vi "GetProperties.vi"(8 "error in":errorcluster, 11 "GObject in":refnum<class "GObject.lvclass">) -> (0 "error out":errorcluster, 3 "GObject out":refnum<class "GObject.lvclass">)   [LabVIEW 2014, in "GObject.lvclass"]
uses:
  GObject.lvclass
  GObject.lvclass/GObject.ctl
  Generic/Generic.lvclass
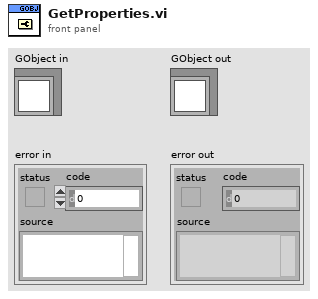
[diagram p1: front panel]
types:
  T1 = typedef "LVBoundsTypeDef.ctl" = cluster{"Width":u32, "Height":u32}
  T2 = typedef "LVRectTypeDef.ctl" = cluster{"Left":i16, "Top":i16, "Right":i16, "Bottom":i16}
  T3 = typedef "LVPositionTypeDef.ctl" = cluster{"Left":i32, "Top":i32}
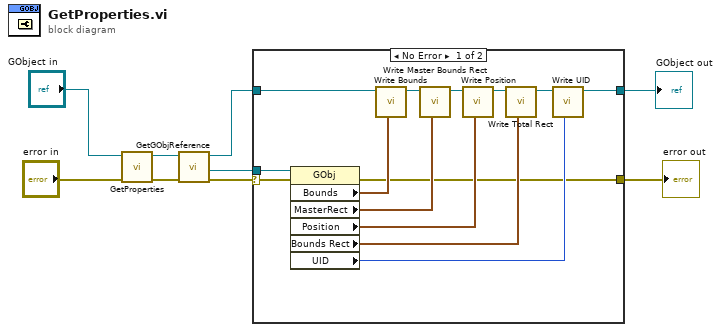
[diagram p0: block diagram]
diagram:
  n1 = call-parent "GetProperties.vi"("error in"="error in", "Generic in"="GObject in") -> ("error out"=w1:errorcluster, "Generic out"=w3:refnum<class "GObject.lvclass">)  [unwired: 8 in]
  n2 = call "GetGObjReference.vi"("error in"=w1, "GObject in"=w3) -> ("error out"=w8:errorcluster, "reference out"=w9:refnum<vi>, "GObject out"=w7:refnum<class "GObject.lvclass">)  [unwired: 5 in]
  n3 = case shown="No Error" w8 {
    selector: w8 -> [w22 w24]
    tunnel: w9 -> [w23 _]
    tunnel: w7 -> [w21 w25]
    tunnel: [w15 w25] -> w6
    tunnel: [w10 w24] -> w5
    frame No Error {
      n4 = property class="GObj"(reference=w23, error in=w22) -> (error out=w10:errorcluster, "Bounds"=w20:T1, "MasterRect"=w14:T2, "Position"=w13:T3, "Bounds Rect"=w12:T2, "UID"=w11:i32)  [unwired: 1 out]
      n5 = call "Write Bounds.vi"("Bounds"=w20, "GObject in"=w21) -> ("GObject out"=w19:refnum<class "GObject.lvclass">)  [unwired: 7 in]
      n6 = call "Write Master Bounds Rect.vi"("Master Bounds Rect"=w14, "GObject in"=w19) -> ("GObject out"=w18:refnum<class "GObject.lvclass">)  [unwired: 7 in]
      n7 = call "Write Position.vi"("Position"=w13, "GObject in"=w18) -> ("GObject out"=w17:refnum<class "GObject.lvclass">)  [unwired: 7 in]
      n8 = call "Write Total Rect.vi"("Total Rect"=w12, "GObject in"=w17) -> ("GObject out"=w16:refnum<class "GObject.lvclass">)  [unwired: 7 in]
      n9 = call "Write UID.vi"("UID"=w11, "GObject in"=w16) -> ("GObject out"=w15:refnum<class "GObject.lvclass">)  [unwired: 7 in]
    }
    frame Error {
    }
  }
  "error out" <- w5
  "GObject out" <- w6
